vi "Test The Class.vi"() -> ()   [LabVIEW 2013, in "PMU Recorder Light.lvlib" / "Statnett C37.118 DLL.lvclass"]
uses:
  Statnett C37.118 DLL.lvclass
  PMU Recorder Light.lvlib
panel:
  out "PMU Status":T1(array[cluster])
  out "React":waveform(dbl)(graph)
  out "Power":waveform(dbl)(graph)
  out "Current":waveform(dbl)(graph)
  out "Voltage":waveform(dbl)(graph)
  out "Frequency Delta":sgl(graph)
  out "PMU Configuration":T2(array[cluster])
  out "Waveform Chart 2":u32(graph)
  out "Frequency":sgl(graph)
  out "New Data?":bool
  out "PDC Configuration":T3
  out "PMU Data":T4(array[cluster])
  out "Time Stamp":timestamp
  in  "Stop":bool
  in  "Wait for Configuration Total Time [ms]":i32=5000
  in  "Wait for Configuration Timeout [ms]":i32=5000
  in  "Boolean 2":bool
  in  "Boolean":bool
  out "error out":errorcluster
  # "TEST"
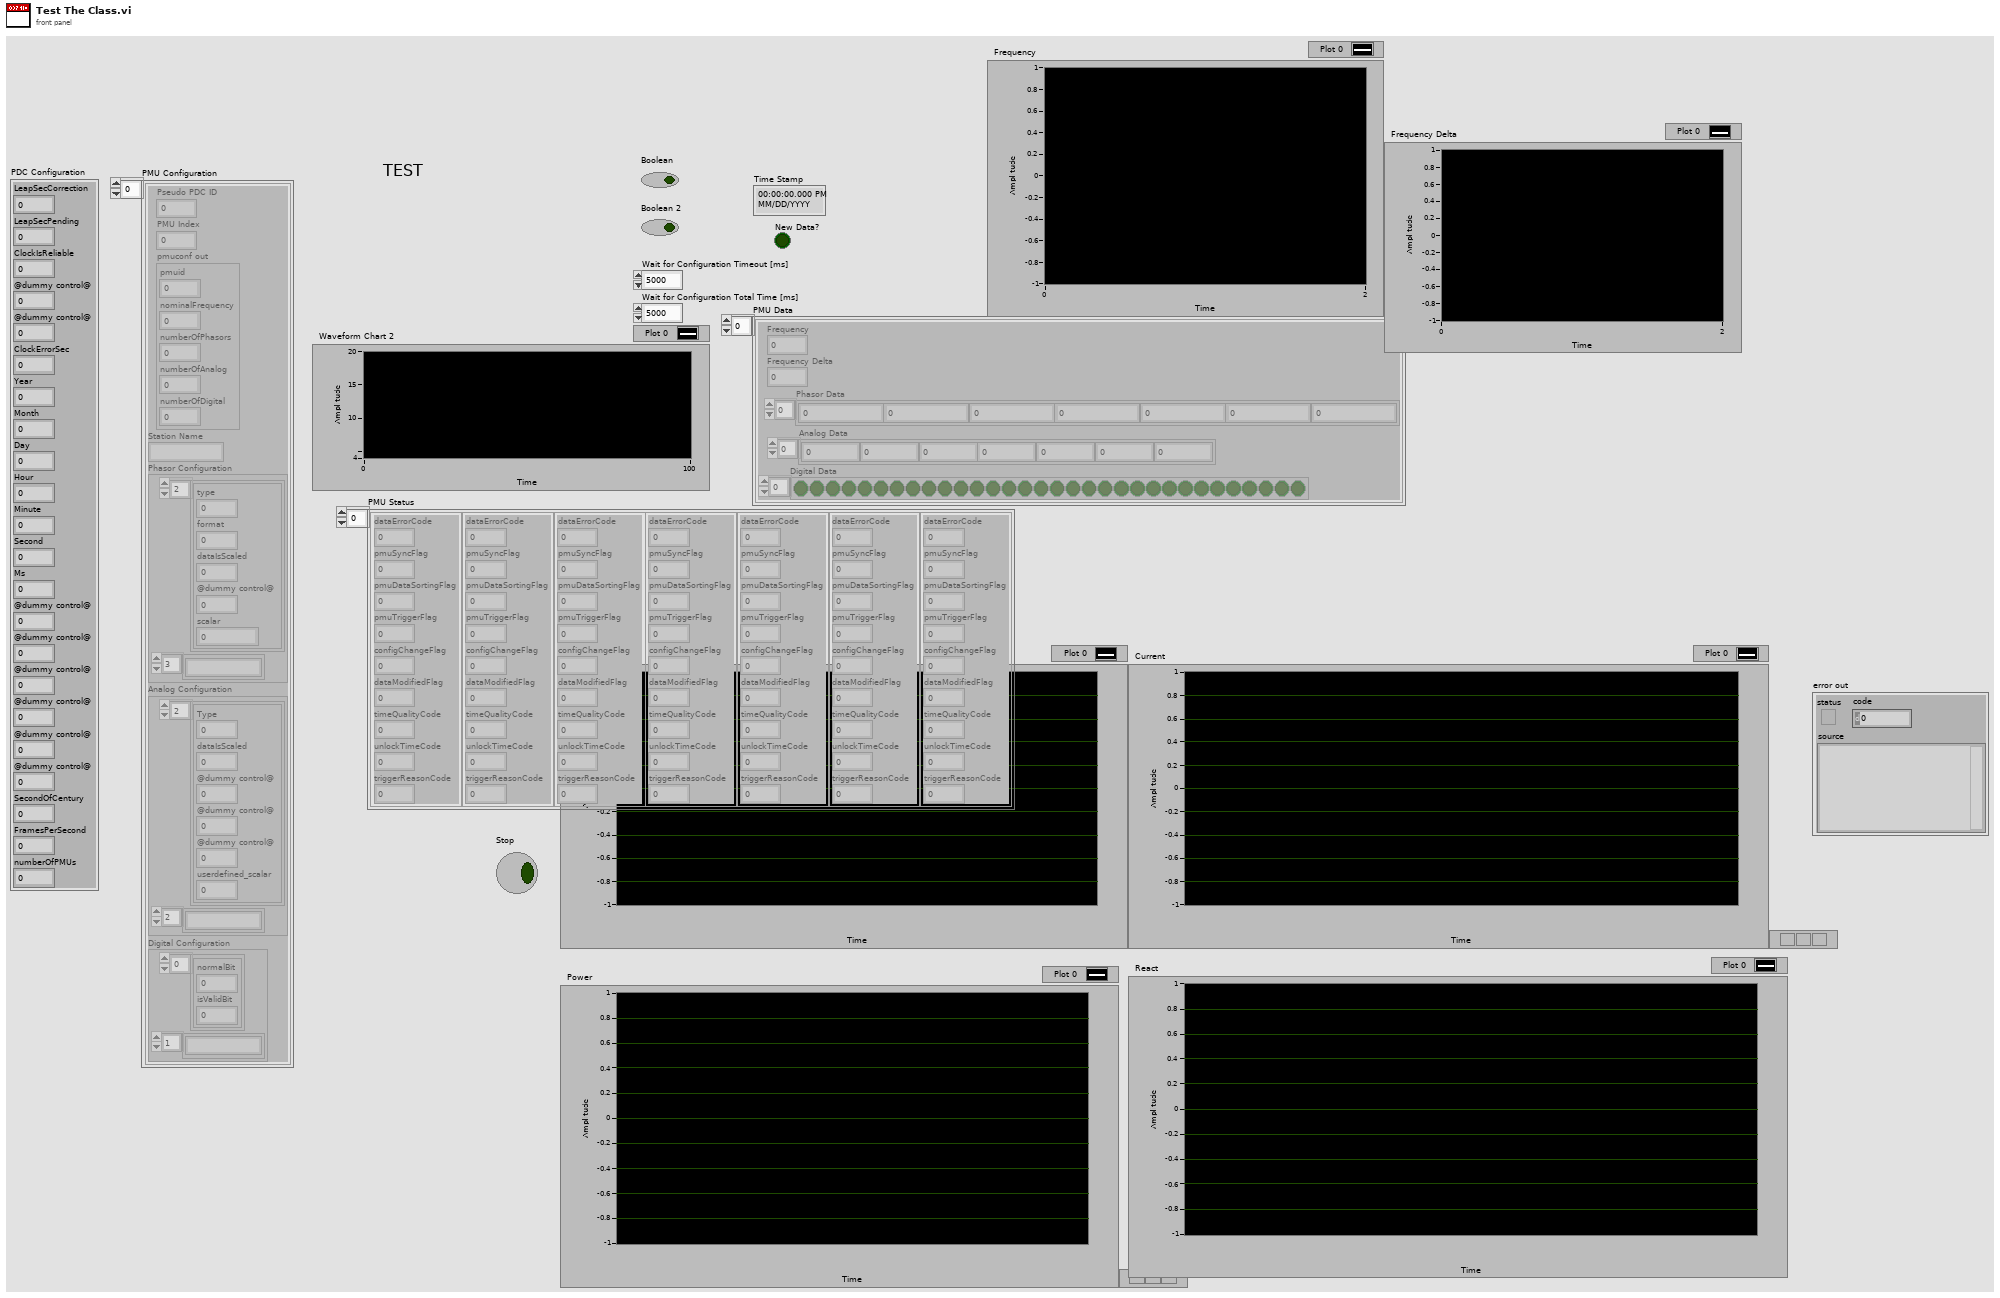
[diagram p1: front panel]
types:
  T1 = cluster{"dataErrorCode":u8, "pmuSyncFlag":u8, "pmuDataSortingFlag":u8, "pmuTriggerFlag":u8, "configChangeFlag":u8, "dataModifiedFlag":u8, "timeQualityCode":u8, "unlockTimeCode":u8, "triggerReasonCode":u8}[]
  T2 = cluster{"Pseudo PDC ID":i32, "PMU Index":i32, "pmuconf out":cluster{"pmuid":i32, "nominalFrequency":sgl, "numberOfPhasors":i32, "numberOfAnalog":i32, "numberOfDigital":i32}, "Station Name":string, "Phasor Configuration":cluster{cluster{"type":u8, "format":u8, "dataIsScaled":u8, "@dummy control@":i8, "scalar":sgl}[], string[]}, "Analog Configuration":cluster{cluster{"Type":i32, "dataIsScaled":u8, "@dummy control@":i8, "@dummy control@":i8, "@dummy control@":i8, "userdefined_scalar":sgl}[], string[]}, "Digital Configuration":cluster{cluster{"normalBit":u8, "isValidBit":u8}[], string[]}}[]
  T3 = cluster{"LeapSecCorrection":i32, "LeapSecPending":u8, "ClockIsReliable":u8, "@dummy control@":i8, "@dummy control@":i8, "ClockErrorSec":sgl, "Year":i16, "Month":i16, "Day":i16, "Hour":i16, "Minute":i16, "Second":i16, "Ms":i16, "@dummy control@":i8, "@dummy control@":i8, "@dummy control@":i8, "@dummy control@":i8, "@dummy control@":i8, "@dummy control@":i8, "SecondOfCentury":dbl, "FramesPerSecond":sgl, "numberOfPMUs":i32}
  T4 = cluster{"Frequency":sgl, "Frequency Delta":sgl, "Phasor Data":csg[], "Analog Data":sgl[], "Digital Data":bool[]}[]
  T5 = cluster{"IP-address":string, "Port":string, "ID Code":u32}
  T6 = cluster{"Frequency":sgl, "Frequency Delta":sgl, "Phasor Data":csg[], "Analog Data":sgl[], "Digital Data":bool[]}
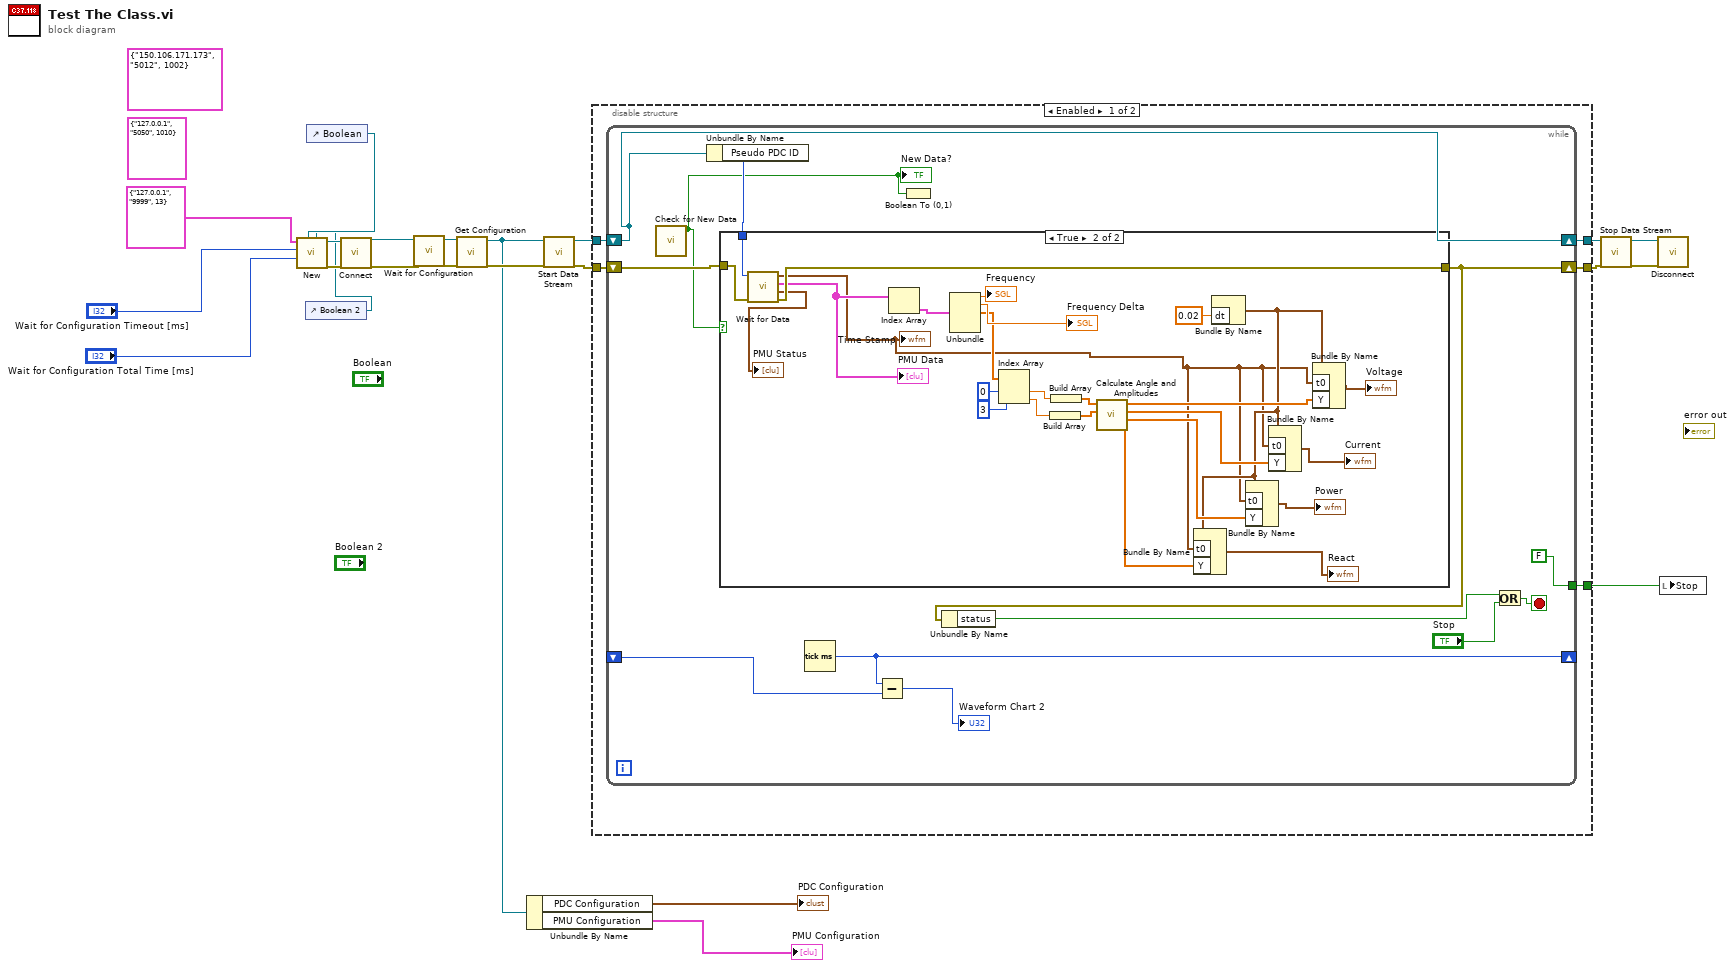
[diagram p0: block diagram]
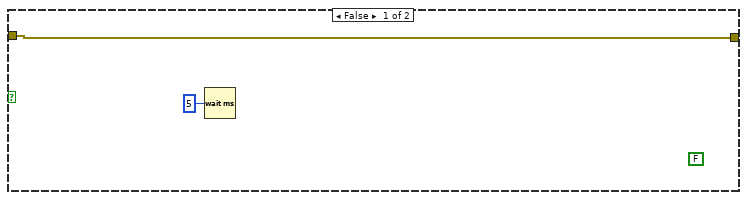
[diagram p2: hidden frame]
diagram:
  (unwired) T5 {"IP-address"="127.0.0.1", "Port"="5050", "ID Code"=1010} ("Connection Settings")
  (unwired) T5 {"IP-address"="150.106.171.173", "Port"="5012", "ID Code"=1002} ("Connection Settings")
  n1 = control-ref of="Boolean 2"() -> (w3:refnum<vi>)
  n2 = control-ref of="Boolean"() -> (w4:refnum<vi>)
  n3 = call "New.vi"("Abort Wait Reference 2"=w3, "Abort Wait Reference"=w4, "Wait for Configuration Total Time [ms]"="Wait for Configuration Total Time [ms]", "Wait for Configuration Timeout [ms]"="Wait for Configuration Timeout [ms]", "Connection Settings"=T5 {"IP-address"="127.0.0.1", "Port"="9999", "ID Code"=13}) -> ("error out"=w21:errorcluster, "Statnett C37.118 DLL out"=w22:refnum<class "Statnett C37.118 DLL.lvclass">)  [unwired: 5 in]
  n4 = call "Connect.vi"("error in (no error)"=w21, "Statnett C37.118 DLL in"=w22) -> ("error out"=w19:errorcluster, "Statnett C37.118 DLL out"=w20:refnum<class "Statnett C37.118 DLL.lvclass">)  [unwired: 8 in]
  n5 = call "Wait for Configuration.vi"("error in (no error)"=w19, "Statnett C37.118 DLL in"=w20) -> ("error out"=w17:errorcluster, "Statnett C37.118 DLL out"=w18:refnum<class "Statnett C37.118 DLL.lvclass">)  [unwired: 8 in]
  n6 = call "Get Configuration.vi"("error in (no error)"=w17, "Statnett C37.118 DLL in"=w18) -> ("error out"=w14:errorcluster, "Statnett C37.118 DLL out"=w6:refnum<class "Statnett C37.118 DLL.lvclass">)  [unwired: 5 in, 3 out]
  n7 = Unbundle By Name(w6) -> ("PDC Configuration"=→"PDC Configuration":T3, "PMU Configuration"=→"PMU Configuration":T2)
  n8 = call "Start Data Stream.vi"("error in (no error)"=w14, "Statnett C37.118 DLL in"=w6) -> ("error out"=w12:errorcluster, "Statnett C37.118 DLL out"=w13:refnum<class "Statnett C37.118 DLL.lvclass">)  [unwired: 8 in]
  n9 = disable-structure shown="Enabled" {
    disable-tunnel: w13 -> [w27 w69]
    disable-tunnel: w12 -> [w26 w68]
    disable-tunnel: [w25 w69] -> w11
    disable-tunnel: [w24 w68] -> w10
    disable-tunnel: [w23 _] -> w7
    frame Enabled {
      n10 = while {
        shift-right: [w29] -> w24
        shift-left: w26 -> [w39]
        shift-right: [w31] -> w25
        shift-left: w27 -> [w31]
        tunnel: [FALSE ("Stop")] -> w23
        shift-right: [w34] -> _
        shift-left: _ -> [w33]
        stop <- w37 stop-if-true
        n11 = call "Check for New Data.vi"() -> ("Data Waiting"=w30:bool)  [unwired: 10 in, 1 out]
        "New Data?" <- w30
        n12 = Unbundle By Name(w31) -> ("Pseudo PDC ID"=w35:i32)
        n13 = case shown="True" w30 {
          tunnel: w39 -> [w41 w67]
          tunnel: [w41 w66] -> w29
          tunnel: w35 -> [_ w65]
          frame False {
            (unwired) FALSE ("status")
            n14 = Wait (ms)(milliseconds to wait=u32 5) -> ()  [unwired: 1 out]
          }
          frame True {
            n15 = call "Wait for Data.vi"("error in (no error)"=w67, "Pseudo PDC ID"=w65) -> ("error out"=w66:errorcluster, "PMU Status"=→"PMU Status":T1, "PMU Data"=w64:T4, "Time Stamp"=w47:timestamp)  [unwired: 3 in, 3 out]
            "Time Stamp" <- w47
            "PMU Data" <- w64
            n16 = Index Array(array=w64) -> (element=w63:T6)  [unwired: 1 in]
            n17 = Unbundle(w63) -> ("Frequency"=→"Frequency":sgl, "Frequency Delta"=→"Frequency Delta":sgl, "Phasor Data"=w60:csg[])  [unwired: 2 out]
            n18 = Index Array(array=w60, index #1=0 ("index"), index #2=3 ("index")) -> (element #1=w57:csg, element #2=w56:csg)
            n19 = Build Array(w56) -> (w54:csg[])
            n20 = Build Array(w57) -> (w55:csg[])
            n21 = call "Calculate Angle and Amplitudes.vi"("Current Phasors"=w54, "Voltage Phasors"=w55) -> ("Reactive Power [MVAR]"=w46:dbl[], "Power [MW]"=w49:dbl[], "Current Amplitude [A]"=w50:dbl[], "Voltage Amplitude [kV]"=w52:dbl[])  [unwired: 5 in, 1 out]
            n22 = Bundle By Name("dt"=0.02) -> (w48:waveform(dbl))  [unwired: 1 in]
            n23 = Bundle By Name(cluster=w48, "t0"=w47, "Y"=w46) -> (→"React":waveform(dbl))
            n24 = Bundle By Name(cluster=w48, "t0"=w47, "Y"=w49) -> (→"Power":waveform(dbl))
            n25 = Bundle By Name(cluster=w48, "t0"=w47, "Y"=w50) -> (→"Current":waveform(dbl))
            n26 = Bundle By Name(cluster=w48, "t0"=w47, "Y"=w52) -> (→"Voltage":waveform(dbl))
          }
        }
        n27 = Tick Count (ms)() -> (millisecond timer value=w34:u32)
        n28 = Subtract(x=w34, y=w33) -> (x-y=→"Waveform Chart 2":u32)
        n29 = Boolean To (0,1)(Boolean=w30) -> ()  [unwired: 1 out]
        n30 = Unbundle By Name(w29) -> ("status"=w28:bool)
        n31 = Or(x=w28, y="Stop") -> (x .or. y?=w37:bool)
      }
    }
    frame Disabled {
    }
  }
  n32 = call "Stop Data Stream.vi"("error in (no error)"=w10, "Statnett C37.118 DLL in"=w11) -> ("error out"=w8:errorcluster, "Statnett C37.118 DLL out"=w9:refnum<class "Statnett C37.118 DLL.lvclass">)  [unwired: 8 in]
  n33 = call "Disconnect.vi"("error in (no error)"=w8, "Statnett C37.118 DLL in"=w9) -> ()  [unwired: 8 in, 2 out]
  n34 = local write "Stop"(w7) -> ()
